vi "initialize.vi"(8 "error in (no error)":errorcluster, 11 "DomeController in":refnum<class "DomeController.lvclass">) -> (0 "error out":errorcluster, 3 "DomeController out":refnum<class "DomeController.lvclass">)   [LabVIEW 2016, in "DomeController.lvclass"]
uses:
  DomeController.lvclass
  DomeController.lvclass/DomeController.ctl
  domeCommunicator/ATDomeCommunicator.lvclass
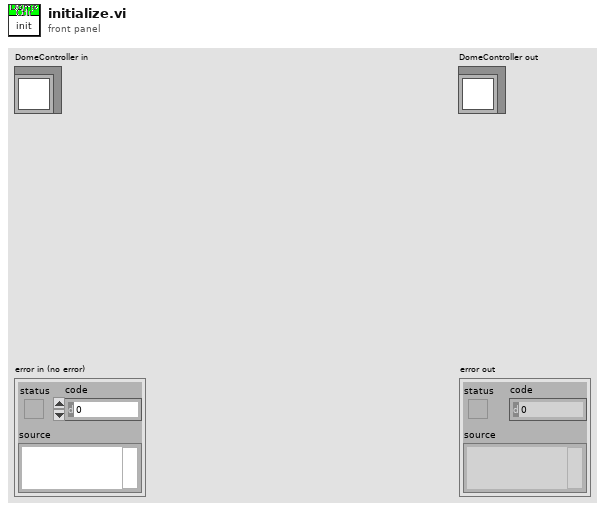
[diagram p1: front panel]
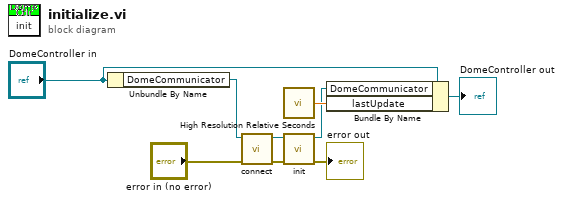
[diagram p0: block diagram]
diagram:
  n1 = Unbundle By Name("DomeController in") -> ("DomeCommunicator"=w9:refnum<class "ATDomeCommunicator.lvclass">)
  n2 = call-dynamic "connect.vi"("error in (no error)"="error in (no error)", "tcpDevice in"=w9) -> ("error out"=w3:errorcluster, "tcpDevice out"=w4:refnum<class "ATDomeCommunicator.lvclass">)  [unwired: 8 in]
  n3 = call <vilib>:"High Resolution Relative Seconds.vi"() -> ("relative seconds"=w5:dbl)
  n4 = call "init.vi"("error in (no error)"=w3, "ATDomeCommunicator in"=w4) -> ("error out"=→"error out":errorcluster, "ATDomeCommunicator out"=w2:refnum<class "ATDomeCommunicator.lvclass">)  [unwired: 8 in]
  n5 = Bundle By Name(cluster="DomeController in", "DomeCommunicator"=w2, "lastUpdate"=w5) -> (→"DomeController out":refnum<class "DomeController.lvclass">)
